vi "Close FPGA.vi"(1 "FPGA in":T1[](array[typedef]) {"UDVs"."To FPGA"."VS ref" format="%.0x"; "UDVs"."From FPGA"."VS ref" format="%.0x"; "VS ref" format="%.0x"; "Output Data"."Output Block Data Refs"."Data Reference" format="%.0x"; "Input Data"."Input Block Data Refs"."Data Reference" format="%.0x"}) -> (0 "FPGA out":T1[](array[typedef]) {"UDVs"."To FPGA"."VS ref" format="%.0x"; "UDVs"."From FPGA"."VS ref" format="%.0x"; "VS ref" format="%.0x"; "Output Data"."Output Block Data Refs"."Data Reference" format="%.0x"; "Input Data"."Input Block Data Refs"."Data Reference" format="%.0x"})   [LabVIEW 2011, in "Scan Engine Custom Device.lvlib"]
uses:
  Scan Engine Custom Device.lvlib
  Type Defs/FPGA Data.ctl
  <vilib>/NI Veristand/Custom Device API/Custom Device Item Ref.ctl
  Type Defs/Input Data.ctl
  <vilib>/NI Veristand/Custom Device API/Block Data Reference.ctl
  <vilib>/NI Veristand/Custom Device API/Data Reference.ctl
  Type Defs/Output Data.ctl
  Type Defs/UDV Data.ctl
  Type Defs/UDV Data Type.ctl
  Type Defs/FXP Config.ctl
  <vilib>/NI Veristand/Custom Device API/Custom Device API.lvlib
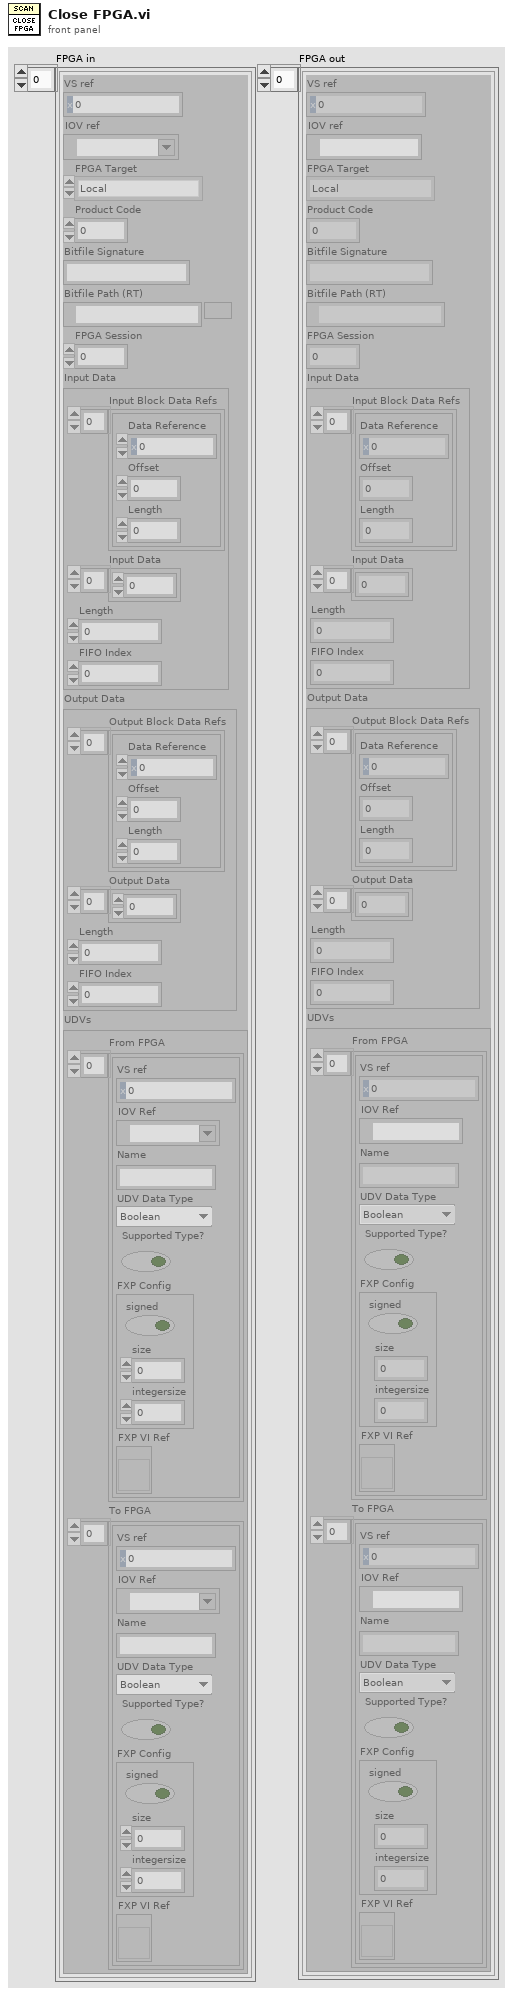
[diagram p1: front panel]
types:
  T1 = typedef "Scan Engine Custom Device.lvlib/FPGA Data.ctl" = cluster{"VS ref":T2, "IOV ref":refnum<k21>, "FPGA Target":enum16{"Local", "EtherCAT"}, "Product Code":u32, "Bitfile Signature":string, "Bitfile Path (RT)":path, "FPGA Session":u32, "Input Data":T3, "Output Data":T6, "UDVs":cluster{"From FPGA":T7[], "To FPGA":T7[]}}
  T2 = typedef "Custom Device API.lvlib/Custom Device Item Ref.ctl" = u64
  T3 = typedef "Scan Engine Custom Device.lvlib/Input Data.ctl" = cluster{"Input Block Data Refs":T4[], "Input Data":dbl[], "Length":i32, "FIFO Index":i32}
  T4 = typedef "Custom Device API.lvlib/Block Data Reference.ctl" = cluster{"Data Reference":T5, "Offset":i32, "Length":i32}
  T5 = typedef "Custom Device API.lvlib/Data Reference.ctl" = i32
  T6 = typedef "Scan Engine Custom Device.lvlib/Output Data.ctl" = cluster{"Output Block Data Refs":T4[], "Output Data":dbl[], "Length":i32, "FIFO Index":i32}
  T7 = typedef "Scan Engine Custom Device.lvlib/UDV Data.ctl" = cluster{"VS ref":T2, "IOV Ref":refnum<k21>, "Name":string, "UDV Data Type":T8, "Supported Type?":bool, "FXP Config":T9, "FXP VI Ref":refnum<vi>}
  T8 = typedef "Scan Engine Custom Device.lvlib/UDV Data Type.ctl" = enum16{"Boolean", "Fixed Point", "Int8", "Int16", "Int32", "Int64", "U32 Bit Field", "UInt8", "UInt16", "UInt32", "UInt64", "Other"}
  T9 = typedef "Scan Engine Custom Device.lvlib/FXP Config.ctl" = cluster{"signed":bool, "size":u32, "integersize":i32}
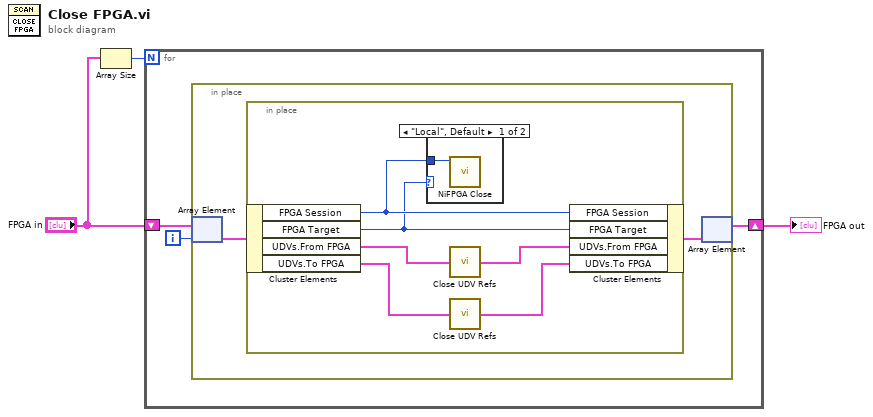
[diagram p0: block diagram]
diagram:
  n1 = Array Size(array="FPGA in") -> (size(s)=w3:i32)
  n2 = for {
    N: w3 -> [_]
    shift-right: [w5] -> w1
    shift-left: "FPGA in" -> [w6]
    i -> [w4]
    n3 = in-place {
      n4 = in-place-array #1(w6, w4) -> (w8:T1)
      n5 = in-place {
        n6 = in-place-cluster #2(w8) -> ("FPGA Session"=w10:u32, "FPGA Target"=w9:enum16{"Local", "EtherCAT"}, "UDVs.From FPGA"=w12:T7[], "UDVs.To FPGA"=w14:T7[])
        n7 = case shown="\"Local\", Default" w9 {
          tunnel: w10 -> [w15 _]
          frame "Local", Default {
            n8 = call "NiFPGA Close.vi"("Session"=w15) -> ()  [unwired: 8 in, 3 out]
          }
          frame "EtherCAT" {
          }
        }
        n9 = call "Close UDV Refs.vi"("UDVs in"=w12) -> ("UDVs out"=w11:T7[])
        n10 = call "Close UDV Refs.vi"("UDVs in"=w14) -> ("UDVs out"=w13:T7[])
        n11 = in-place-cluster #2("FPGA Session"=w10, "FPGA Target"=w9, "UDVs.From FPGA"=w11, "UDVs.To FPGA"=w13) -> (w7:T1)
      }
      n12 = in-place-array #1(w7) -> (w5:T1[])  [unwired: 1 out]
    }
  }
  "FPGA out" <- w1
